vi "Flow Curve Test SM.vi"() -> ()   [LabVIEW 2013]
uses:
  Type Definitions/EquipReferences.ctl
  Type Definitions/Intellfaucet Mode.ctl
  Type Definitions/ChannelSettings.ctl
  <vilib>/Analysis/baseanly.llb/Mean (DBL).vi
  <vilib>/Utility/config.llb/Write Key (String).vi
  <vilib>/Utility/config.llb/NI_LVConfig.lvlib
  <vilib>/Analysis/NI_AALBase.lvlib
panel:
  in  "Temperature(F)":dbl(slide)=58.0 scale=40.0..120.0
  out "Sample":i32
  in  "Sample Delay":u32=500
  in  "Init Delay":u32=5000
  out "Save Triger":i32
  in  "Config File Path":path=path "C:/work/flowconfig.ini"
  out "Percent Input":dbl
  in  "Number of Samples":i32=30
  out "Flow":dbl
  out "Flowrate":dbl(graph)
  out "Results(Flow,Percent)":dbl[][](array[numeric])
  in  "Percent Open Test Data":dbl[](array[numeric])=[0.0, 15.0, 18.0, 20.0, 25.0, 30.0, 35.0, 40.0, 50.0, 60.0, 70.0, 80.0, 90.0, 100.0]
  in  "Equipment":T1={"MW100"="COM1", "AG34970"="MW100", "Chamber"="A-34972A"}
  in  "Semiphore":T2
  out "Error Out":errorcluster
  in  "Error In":errorcluster
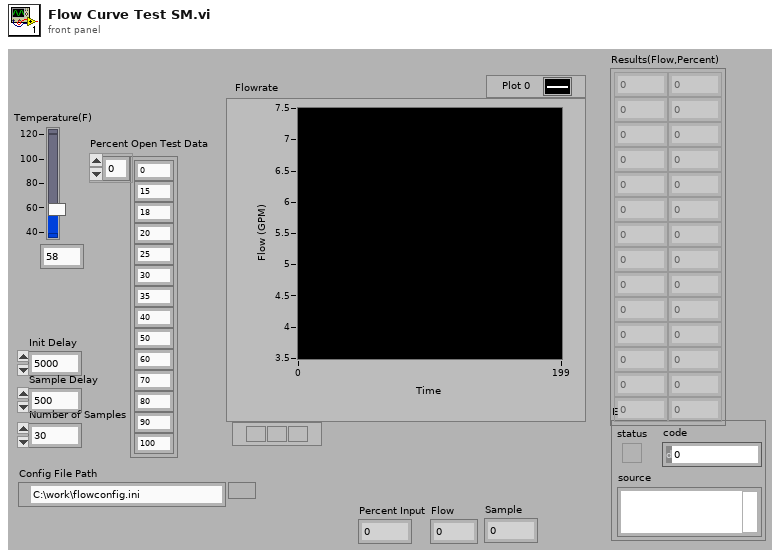
[diagram p1: front panel]
types:
  T1 = typedef "EquipReferences.ctl" = cluster{"MW100":refnum<visa-resource-name>, "AG34970":refnum<visa-resource-name>, "Chamber":refnum<visa-resource-name>}
  T2 = typedef "Semaphore RefNum" = refnum<k1>
  T3 = typedef "Intellfaucet Mode.ctl" = enum16{"Adjust Temp", "Adjust Flow", "Start Flow", "Stop Flow"}
  T4 = typedef "NI_LVConfig.lvlib/Config Data RefNum.ctl" = refnum<k1>
  T5 = typedef "ChannelSettings.ctl" = u32
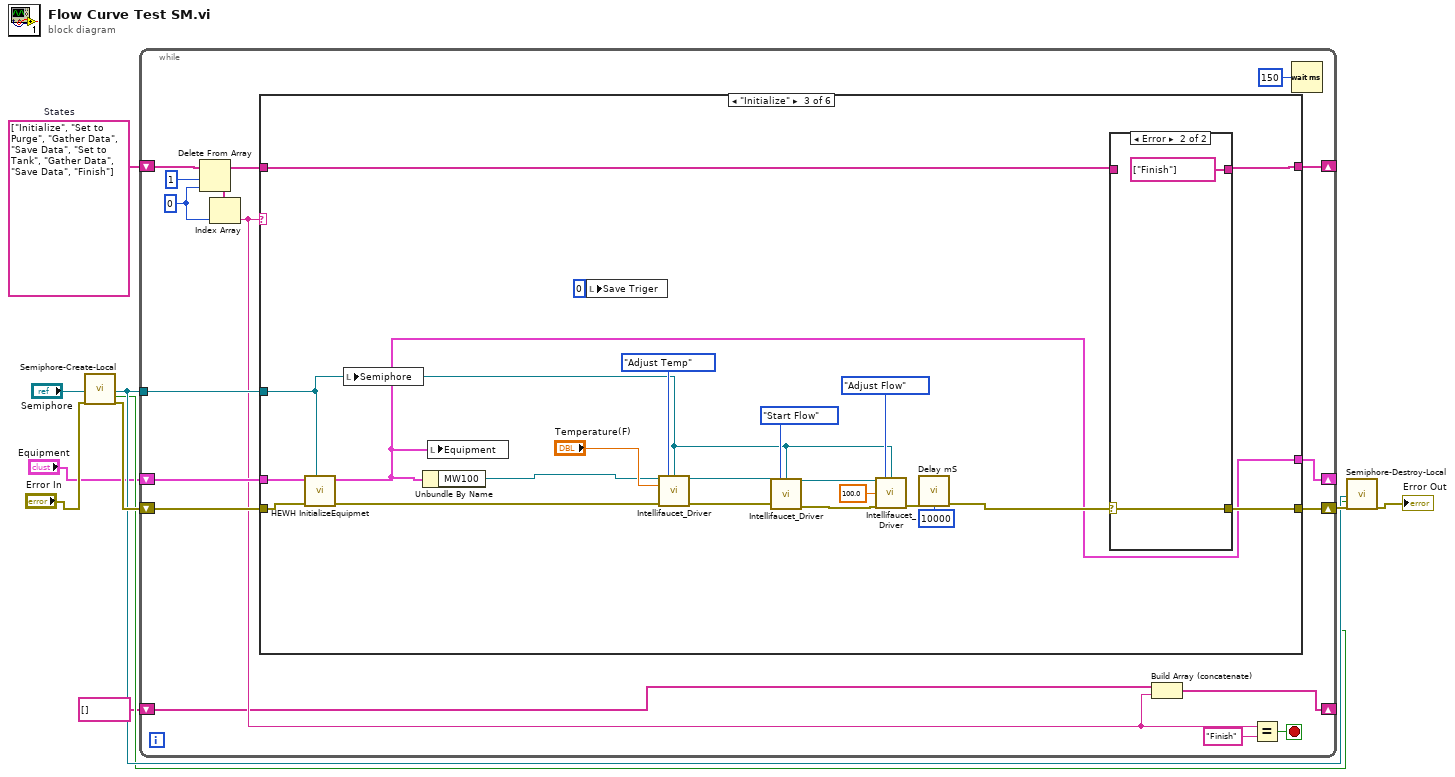
[diagram p0: block diagram]
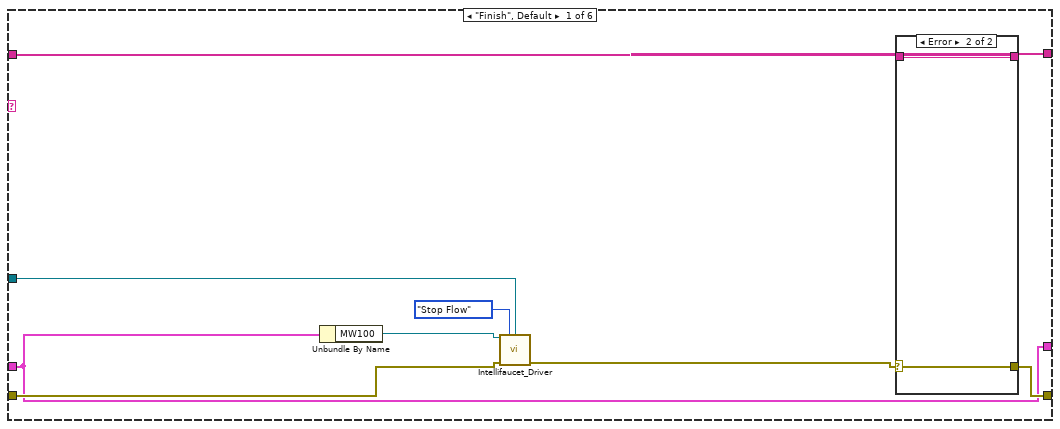
[diagram p2: hidden frame]
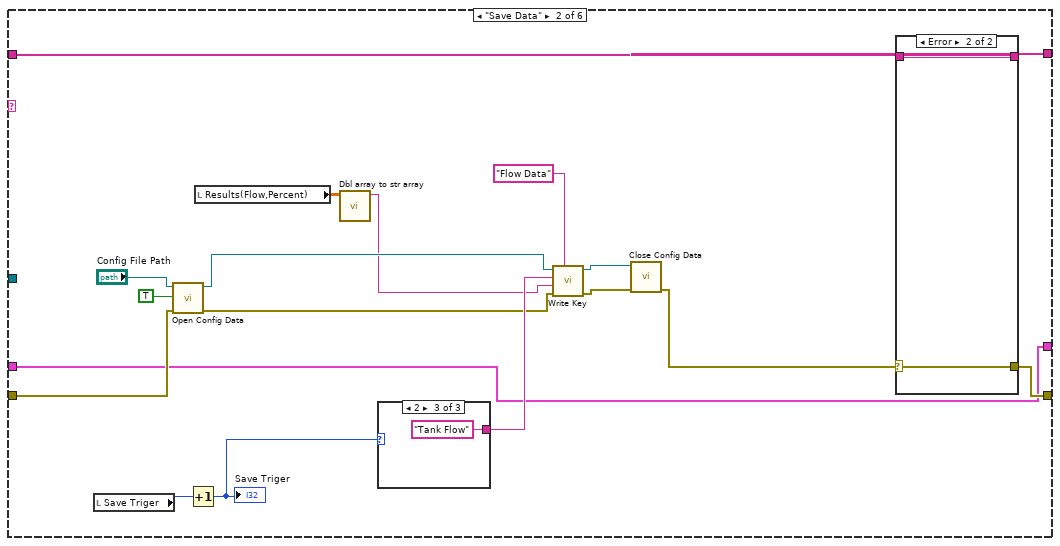
[diagram p4: hidden frame]
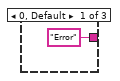
[diagram p5: hidden frame]
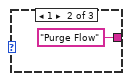
[diagram p6: hidden frame]
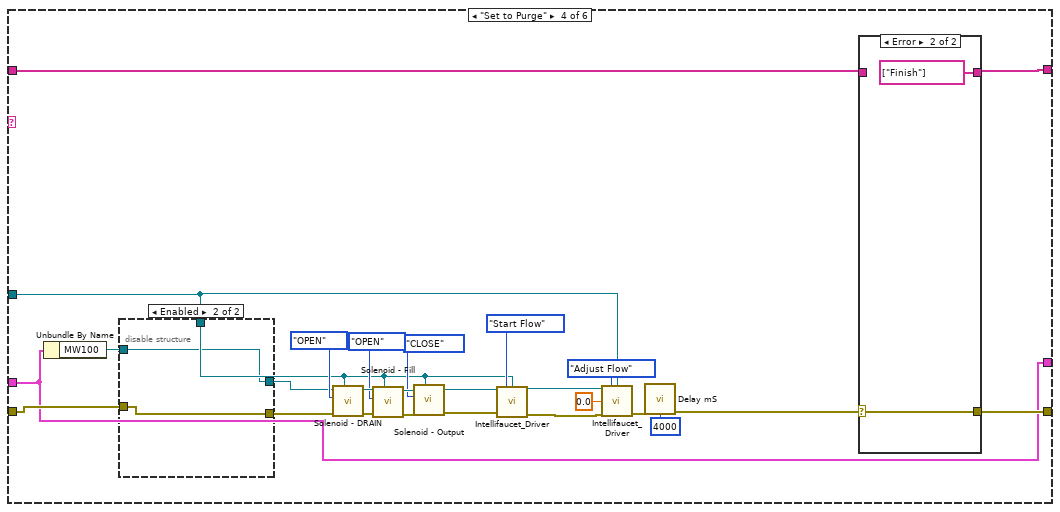
[diagram p9: hidden frame]
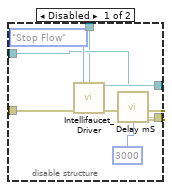
[diagram p10: hidden frame]
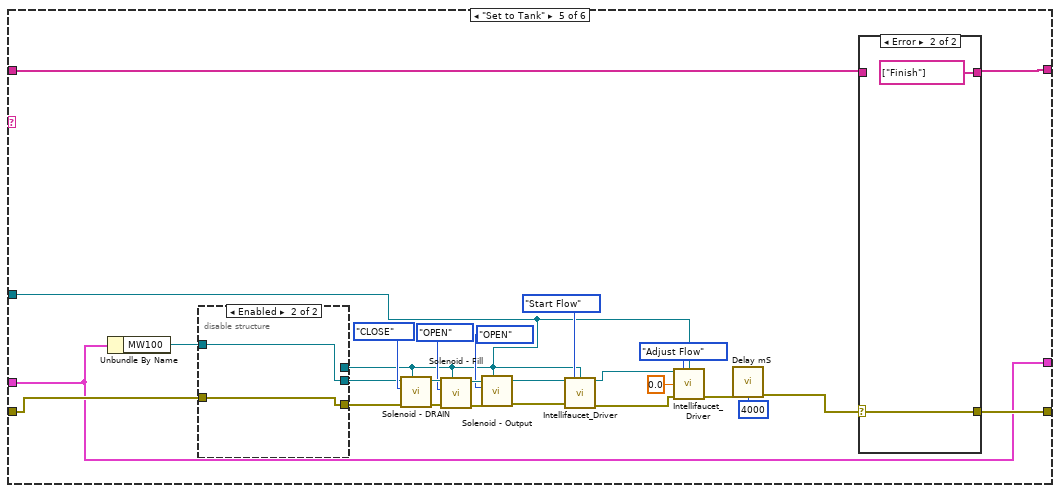
[diagram p12: hidden frame]
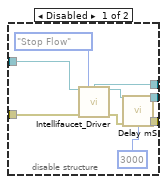
[diagram p13: hidden frame]
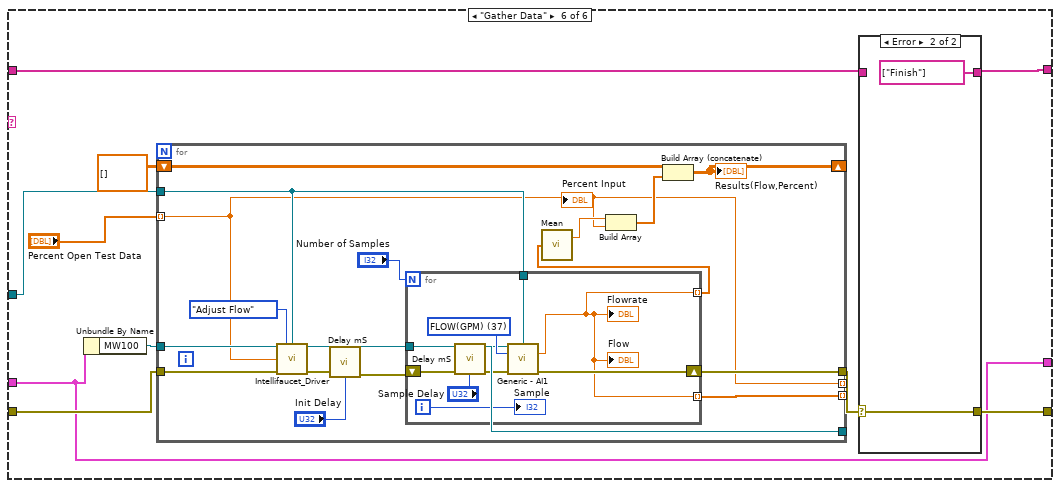
[diagram p15: hidden frame]
diagram:
  w10 = string[] ["Initialize", "Set to Purge", "Gather Data", "Save Data", "Set to Tank", "Gather Data", "Save Data", "Finish"]  # States
  n1 = call "Semiphore-Create-Local.vi"("Semiphore"="Semiphore", "error in (no error)"="Error In") -> ("semaphore"=w4:T2, "Local?"=w3:bool, "error out"=w7:errorcluster)  [unwired: 15 in]
  n2 = while {
    shift-right: [w23] -> _
    shift-left: w10 -> [w27]
    shift-right: [w20] -> w6
    shift-left: w7 -> [w19]
    tunnel: w4 -> [w16]
    shift-right: [w12] -> _
    shift-left: string[] [] -> [w13]
    shift-right: [w11] -> _
    shift-left: "Equipment" -> [w15]
    stop <- w18 stop-if-true
    w24 = 0 ("index")
    n3 = Delete From Array(array=w27, length=1, index=w24) -> (deleted portion=w25:string[], array with subset deleted=w22:string[])
    n4 = Index Array(array=w25, index=w24) -> (element=w14:string)
    n5 = case shown="\"Initialize\"" w14 {
      tunnel: [w36 w58 w82 w114 w154 w178] -> w23
      tunnel: w22 -> [w35 w57 w83 w115 w155 w179]
      tunnel: [w34 w56 w84 w116 w156 w180] -> w20
      tunnel: w19 -> [w33 w47 w86 w101 w141 w176]
      tunnel: w16 -> [w29 _ w66 w92 w135 w173]
      tunnel: w15 -> [w31 w41 w85 w91 w131 w171]
      tunnel: [w31 w41 w72 w91 w131 w171] -> w11
      frame "Finish", Default {
        n6 = Unbundle By Name(w31) -> ("MW100"=w30:refnum<visa-resource-name>)
        n7 = call "Intellifaucet_Driver.vi"("VISA session"=w30, "Mode"=Intellfaucet_Mode."Stop Flow", "Semiphore"=w29, "Error In"=w33) -> ("Error Out"=w32:errorcluster)  [unwired: 10 in, 1 out]
        n8 = case shown="Error" w32 {
          selector: w32 -> [w37 w39]
          tunnel: [w38 w40] -> w36
          tunnel: w35 -> [w38 w40]
          tunnel: [w37 w39] -> w34
          frame No Error {
          }
          frame Error {
          }
        }
      }
      frame "Save Data" {
        n9 = local read "Save Triger"() -> (w42:i32)
        n10 = call <vilib>:"Open Config Data.vi"("error in (no error)"=w47, "create file if necessary (T)"=TRUE, "configuration file path"="Config File Path") -> ("error out"=w50:errorcluster, "refnum"=w52:T4)  [unwired: 7 out]
        n11 = Increment(x=w42) -> (x+1=w43:i32)
        "Save Triger" <- w43
        n12 = local read "Results(Flow,Percent)"() -> (w55:dbl[][])
        n13 = call "Dbl array to str array.vi"("Array in"=w55) -> ("String array out"=w44:string)  [unwired: 9 in, 1 out]
        n14 = case shown="2" w43 {
          tunnel: ["Error" ("key") "Purge Flow" ("key") "Tank Flow" ("key")] -> w51
          frame 0, Default {
          }
          frame 1 {
          }
          frame 2 {
          }
        }
        n15 = call-poly <vilib>:"Write Key.vi"("section"="Flow Data", "error in (no error)"=w50, "value"=w44, "key"=w51, "refnum"=w52) -> ("error out"=w49:errorcluster, "refnum out"=w48:T4)  [unwired: 1 in, 4 out]
        n16 = call <vilib>:"Close Config Data.vi"("error in (no error)"=w49, "refnum"=w48) -> ("error out"=w46:errorcluster)  [unwired: 1 in, 8 out]
        n17 = case shown="Error" w46 {
          selector: w46 -> [w62 w64]
          tunnel: [w63 w65] -> w58
          tunnel: w57 -> [w63 w65]
          tunnel: [w62 w64] -> w56
          frame No Error {
          }
          frame Error {
          }
        }
      }
      frame "Initialize" {
        n18 = call "HEWH InitializeEquipmet.vi"("Semiphore"=w66, "Error In"=w86, "Equipment"=w85) -> ("Error Out"=w69:errorcluster, "Equipment Out"=w72:T1)  [unwired: 5 in, 2 out]
        n19 = local write "Semiphore"(w66) -> ()
        n20 = Unbundle By Name(w72) -> ("MW100"=w67:refnum<visa-resource-name>)
        n21 = local write "Equipment"(w72) -> ()
        n22 = local write "Save Triger"(0 ("Save Triger")) -> ()
        n23 = call "Intellifaucet_Driver.vi"("VISA session"=w67, "Mode"=Intellfaucet_Mode."Adjust Temp", "Semiphore"=w66, "Temperature(F)"="Temperature(F)", "Error In"=w69) -> ("Error Out"=w68:errorcluster)  [unwired: 9 in, 1 out]
        n24 = call "Intellifaucet_Driver.vi"("VISA session"=w67, "Mode"=Intellfaucet_Mode."Start Flow", "Semiphore"=w66, "Error In"=w68) -> ("VISA session out"=w74:refnum<visa-resource-name>, "Error Out"=w75:errorcluster)  [unwired: 10 in]
        n25 = call "Intellifaucet_Driver.vi"("VISA session"=w74, "Mode"=Intellfaucet_Mode."Adjust Flow", "Semiphore"=w66, "Percent Flow"=100.0, "Error In"=w75) -> ("Error Out"=w77:errorcluster)  [unwired: 9 in, 1 out]
        n26 = call "Delay mS.vi"("Error In"=w77, "milliseconds to wait"=u32 10000) -> ("Error Out"=w73:errorcluster)  [unwired: 13 in]
        n27 = case shown="Error" w73 {
          selector: w73 -> [w87 w90]
          tunnel: [w88 string[] ["Finish"] ("States")] -> w82
          tunnel: w83 -> [w88 _]
          tunnel: [w87 w90] -> w84
          frame No Error {
          }
          frame Error {
          }
        }
      }
      frame "Set to Purge" {
        n28 = Unbundle By Name(w91) -> ("MW100"=w100:refnum<visa-resource-name>)
        n29 = disable-structure shown="Enabled" {
          disable-tunnel: [w124 w126] -> w105
          disable-tunnel: [w122 w125] -> w104
          disable-tunnel: w101 -> [w119 w125]
          disable-tunnel: w100 -> [w118 w126]
          disable-tunnel: w92 -> [w117 _]
          frame Disabled {
            n30 = call "Intellifaucet_Driver.vi"("VISA session"=w118, "Mode"=Intellfaucet_Mode."Stop Flow", "Semiphore"=w117, "Error In"=w119) -> ("VISA session out"=w124:refnum<visa-resource-name>, "Error Out"=w123:errorcluster)  [unwired: 10 in]
            n31 = call "Delay mS.vi"("Error In"=w123, "milliseconds to wait"=u32 3000) -> ("Error Out"=w122:errorcluster)  [unwired: 13 in]
          }
          frame Enabled {
          }
        }
        n32 = call "Solenoid - DRAIN.vi"("Semiphore"=w92, "Error In"=w104, "VALVE OPEN CLOSE"=enum8{"OPEN", "CLOSE"}."OPEN", "VISA session"=w105) -> ("Error Out"=w113:errorcluster, "dup VISA session"=w112:refnum<visa-resource-name>)  [unwired: 6 in]
        n33 = call "Solenoid - Fill.vi"("Semiphore"=w92, "Error In"=w113, "VALVE OPEN CLOSE"=enum8{"OPEN", "CLOSE"}."OPEN" ("OPEN CLOSE"), "VISA session"=w112) -> ("Error Out"=w110:errorcluster, "dup VISA session"=w109:refnum<visa-resource-name>)  [unwired: 6 in]
        n34 = call "Solenoid - Output.vi"("Semiphore"=w92, "Error In"=w110, "OPEN CLOSE"=enum8{"CLOSE", "OPEN"}."CLOSE", "VISA session"=w109) -> ("Error Out"=w102:errorcluster, "dup VISA session"=w106:refnum<visa-resource-name>)  [unwired: 6 in]
        n35 = call "Intellifaucet_Driver.vi"("VISA session"=w106, "Mode"=Intellfaucet_Mode."Start Flow", "Semiphore"=w92, "Error In"=w102) -> ("VISA session out"=w93:refnum<visa-resource-name>, "Error Out"=w95:errorcluster)  [unwired: 10 in]
        n36 = call "Intellifaucet_Driver.vi"("VISA session"=w93, "Mode"=Intellfaucet_Mode."Adjust Flow", "Semiphore"=w92, "Percent Flow"=0.0, "Error In"=w95) -> ("Error Out"=w97:errorcluster)  [unwired: 9 in, 1 out]
        n37 = call "Delay mS.vi"("Error In"=w97, "milliseconds to wait"=u32 4000) -> ("Error Out"=w94:errorcluster)  [unwired: 13 in]
        n38 = case shown="Error" w94 {
          selector: w94 -> [w127 w130]
          tunnel: [w128 string[] ["Finish"] ("States")] -> w114
          tunnel: w115 -> [w128 _]
          tunnel: [w127 w130] -> w116
          frame No Error {
          }
          frame Error {
          }
        }
      }
      frame "Set to Tank" {
        n39 = Unbundle By Name(w131) -> ("MW100"=w140:refnum<visa-resource-name>)
        n40 = disable-structure shown="Enabled" {
          disable-tunnel: [w164 w165] -> w145
          disable-tunnel: [w162 w166] -> w144
          disable-tunnel: w141 -> [w159 w166]
          disable-tunnel: w140 -> [w158 w165]
          disable-tunnel: w135 -> [w157 _]
          frame Disabled {
            n41 = call "Intellifaucet_Driver.vi"("VISA session"=w158, "Mode"=Intellfaucet_Mode."Stop Flow", "Semiphore"=w157, "Error In"=w159) -> ("VISA session out"=w164:refnum<visa-resource-name>, "Error Out"=w163:errorcluster)  [unwired: 10 in]
            n42 = call "Delay mS.vi"("Error In"=w163, "milliseconds to wait"=u32 3000) -> ("Error Out"=w162:errorcluster)  [unwired: 13 in]
          }
          frame Enabled {
          }
        }
        n43 = call "Solenoid - DRAIN.vi"("Semiphore"=w135, "Error In"=w144, "VALVE OPEN CLOSE"=enum8{"OPEN", "CLOSE"}."CLOSE", "VISA session"=w145) -> ("Error Out"=w153:errorcluster, "dup VISA session"=w152:refnum<visa-resource-name>)  [unwired: 6 in]
        n44 = call "Solenoid - Fill.vi"("Semiphore"=w135, "Error In"=w153, "VALVE OPEN CLOSE"=enum8{"OPEN", "CLOSE"}."OPEN" ("OPEN CLOSE"), "VISA session"=w152) -> ("Error Out"=w150:errorcluster, "dup VISA session"=w149:refnum<visa-resource-name>)  [unwired: 6 in]
        n45 = call "Solenoid - Output.vi"("Semiphore"=w135, "Error In"=w150, "OPEN CLOSE"=enum8{"CLOSE", "OPEN"}."OPEN", "VISA session"=w149) -> ("Error Out"=w142:errorcluster, "dup VISA session"=w146:refnum<visa-resource-name>)  [unwired: 6 in]
        n46 = call "Intellifaucet_Driver.vi"("VISA session"=w146, "Mode"=Intellfaucet_Mode."Start Flow", "Semiphore"=w135, "Error In"=w142) -> ("VISA session out"=w136:refnum<visa-resource-name>, "Error Out"=w137:errorcluster)  [unwired: 10 in]
        n47 = call "Intellifaucet_Driver.vi"("VISA session"=w136, "Mode"=Intellfaucet_Mode."Adjust Flow", "Semiphore"=w135, "Percent Flow"=0.0, "Error In"=w137) -> ("Error Out"=w134:errorcluster)  [unwired: 9 in, 1 out]
        n48 = call "Delay mS.vi"("Error In"=w134, "milliseconds to wait"=u32 4000) -> ("Error Out"=w133:errorcluster)  [unwired: 13 in]
        n49 = case shown="Error" w133 {
          selector: w133 -> [w167 w170]
          tunnel: [w168 string[] ["Finish"] ("States")] -> w154
          tunnel: w155 -> [w168 _]
          tunnel: [w167 w170] -> w156
          frame No Error {
          }
          frame Error {
          }
        }
      }
      frame "Gather Data" {
        n50 = Unbundle By Name(w171) -> ("MW100"=w177:refnum<visa-resource-name>)
        n51 = for {
          tunnel: [w193] -> _ mode=indexing
          tunnel: w176 -> [w196]
          tunnel: w173 -> [w195]
          tunnel: [w181] -> _ mode=indexing
          tunnel: [w197] -> w175
          tunnel: "Percent Open Test Data" -> [w181] mode=indexing
          tunnel: [w192] -> _
          tunnel: w177 -> [w191]
          shift-right: [w187] -> _
          shift-left: dbl[][] [] -> [w186]
          n52 = call "Intellifaucet_Driver.vi"("VISA session"=w191, "Mode"=Intellfaucet_Mode."Adjust Flow", "Semiphore"=w195, "Percent Flow"=w181, "Error In"=w196) -> ("VISA session out"=w192:refnum<visa-resource-name>, "Error Out"=w185:errorcluster)  [unwired: 9 in]
          n53 = call "Delay mS.vi"("Error In"=w185, "milliseconds to wait"="Init Delay") -> ("Error Out"=w184:errorcluster)  [unwired: 13 in]
          n54 = for {
            N: "Number of Samples" -> [_]
            tunnel: w195 -> [w202]
            tunnel: [w199] -> w193 mode=indexing
            tunnel: w192 -> [w201]
            shift-right: [w204] -> w197
            shift-left: w184 -> [w203]
            tunnel: [w199] -> w190 mode=indexing
            i -> [w198]
            w206 = T5 37 items=["4-20_OUT", "Pres_HI1", "Pres_HI2", "Pres_LOW", "Pres_PIN", "HEATER_TOP", "HEATER_BOT", "T_Shell", "FLOWMETER", "WATT_SENSE", "WH_TICK", "Tc_1", "Tc_2", "Tc_3", "Tc_4", "Tc_5", "Tc_6", "Tc_down", "T_Shell_2", "T_Shell_3", "T_Shell_4", "RTD_IN", "RTD_OUT", "RTD_AMB", "INTF_TEMPFLO", "INTF_READY", "INTF_START", "INTF_STOP", "DRM_LOW", "DRM_HIGH", "PWR_MAIN", "VLV_DUMP", "VLV_OUT", "VLV_IN", "WATT_HOURS", "FLOW(SAMPLE)", "GALLONS", "FLOW(GPM)"] ("Channel_Enum")
            n55 = call "Delay mS.vi"("Error In"=w203, "milliseconds to wait"="Sample Delay") -> ("Error Out"=w205:errorcluster)  [unwired: 13 in]
            n56 = call "Generic - AI1.vi"("MW100"=w201, "Semiphore"=w202, "Channel_Enum"=w206, "Error In"=w205) -> ("Value"=w199:dbl, "Error Out"=w204:errorcluster)  [unwired: 9 in, 1 out]
            "Flow" <- w199
            "Flowrate" <- w199
            "Sample" <- w198
          }
          n57 = call-poly <vilib>:"Mean.vi"("X"=w190) -> ("mean"=w188:dbl)  [unwired: 1 out]
          n58 = Build Array(w188, w181) -> (w189:dbl[])
          n59 = Build Array (concatenate)(w186, w189) -> (w187:dbl[][])
          "Results(Flow,Percent)" <- w187
          "Percent Input" <- w181
        }
        n60 = case shown="Error" w175 {
          selector: w175 -> [w207 w210]
          tunnel: [w208 string[] ["Finish"] ("States")] -> w178
          tunnel: w179 -> [w208 _]
          tunnel: [w207 w210] -> w180
          frame No Error {
          }
          frame Error {
          }
        }
      }
    }
    n61 = Build Array (concatenate)(w13, w14) -> (w12:string[])
    n62 = Equal?(x=w14, y="Finish") -> (x = y?=w18:bool)
    n63 = Wait (ms)(milliseconds to wait=u32 150) -> ()  [unwired: 1 out]
  }
  n64 = call "Semiphore-Destroy-Local.vi"("Semiphore"=w4, "Local?"=w3, "error in (no error)"=w6) -> ("error out"=→"Error Out":errorcluster)  [unwired: 16 in]
